vi "Check Caller.vi"(8 "error in (no error)":errorcluster, 11 "WorkSpace / Repo path":path) -> (0 "error out":errorcluster)   [LabVIEW 2019]
panel:
  out "Array 3":string[][](array[string])
  out "All Files in Dir":path[](array[path])
  out "Array":path[][](array[path])
  in  "Scan":bool
  in  "Status":string
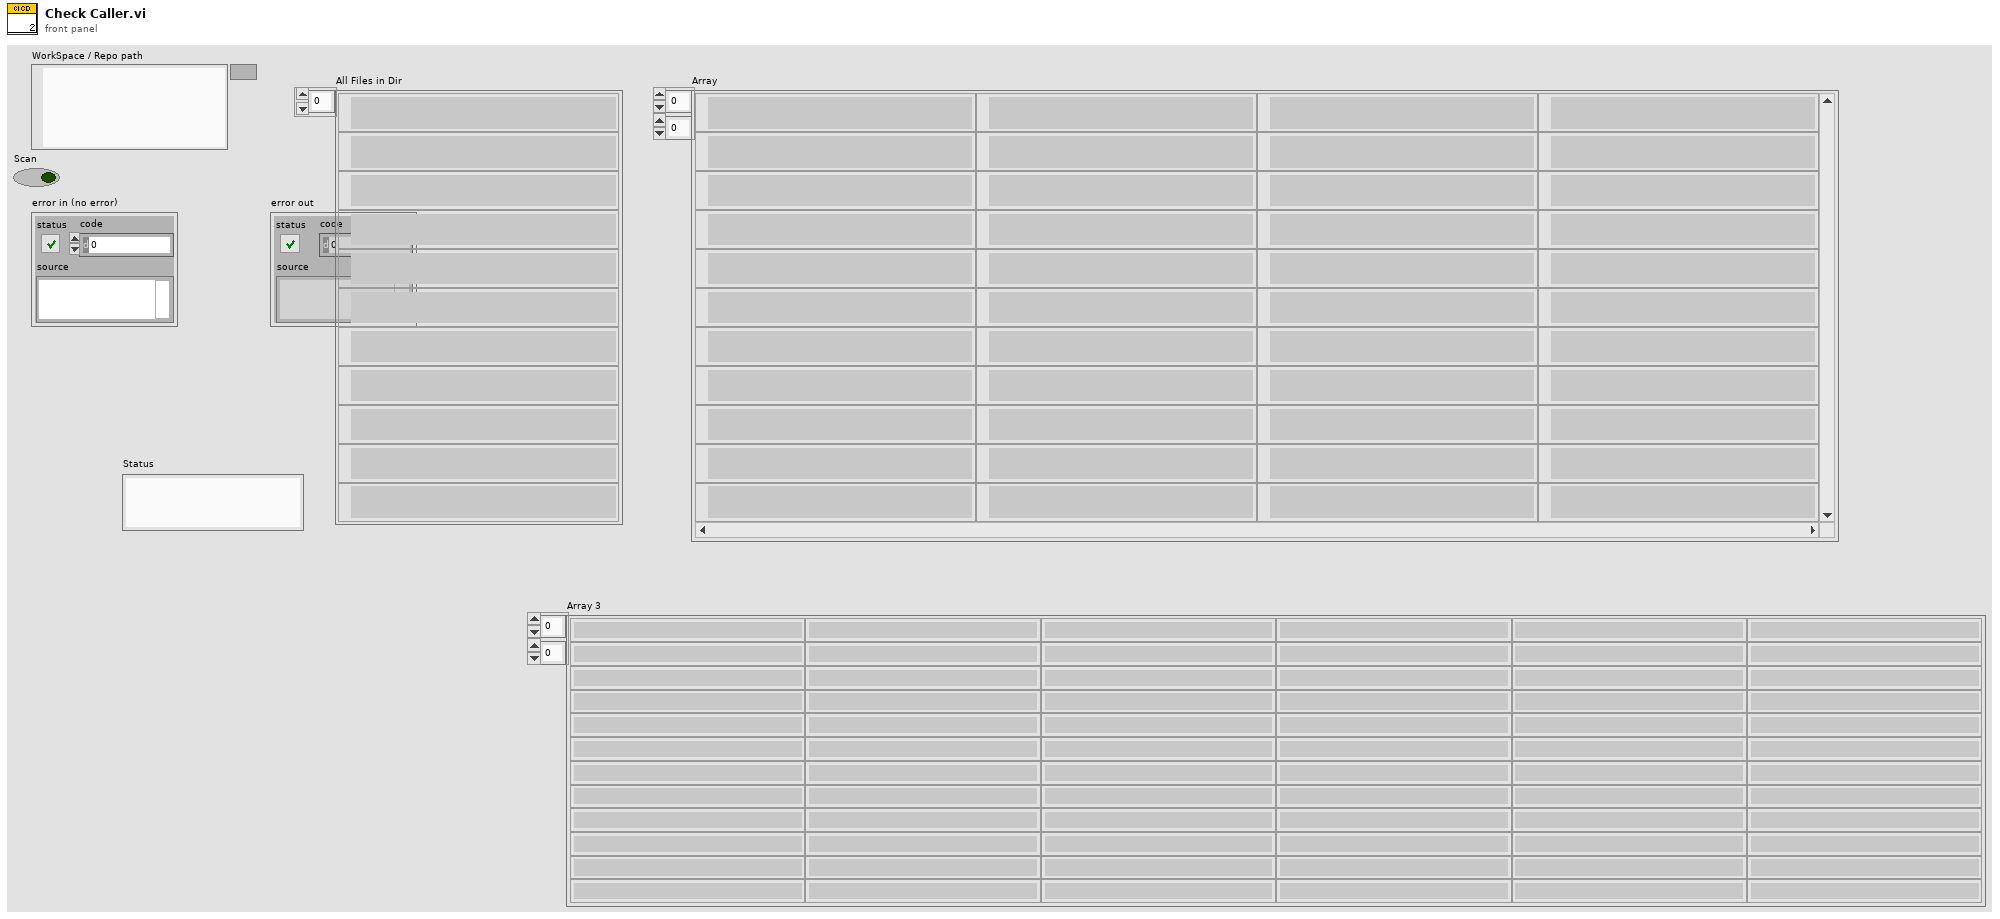
[diagram p1: front panel]
types:
  T1 = enum16{"open", "replace", "create", "open or create", "replace or create", "replace or create with confirmation"}
  T2 = typedef "NI_FileType.lvlib/LVFileType.ctl" = enum32{"Invalid file", "Unknown type", "Instrument", "Control", "Polymorphic VI", "Project", "Library", "LVClass", "XControl", "XNode", "Shared library", ".NET assembly", "ActiveX interface", "CIN", "Run-time menu", "Palette menu", "Help file", "LLB", "XNode Edit Dependency", "Class Private Data Control", "Statechart", "MathScript .m file", "Ladder Diagram", "LVLibp", "XNode Build Dependency"}
  T3 = cluster{"path":path, "delimited name":string, "type":T2, "iState":u32, "iStyle":u16, "wStyle":u16, "buttons":u16, "viflags":u32, "viflags2":u32, "links":u32[]}[]
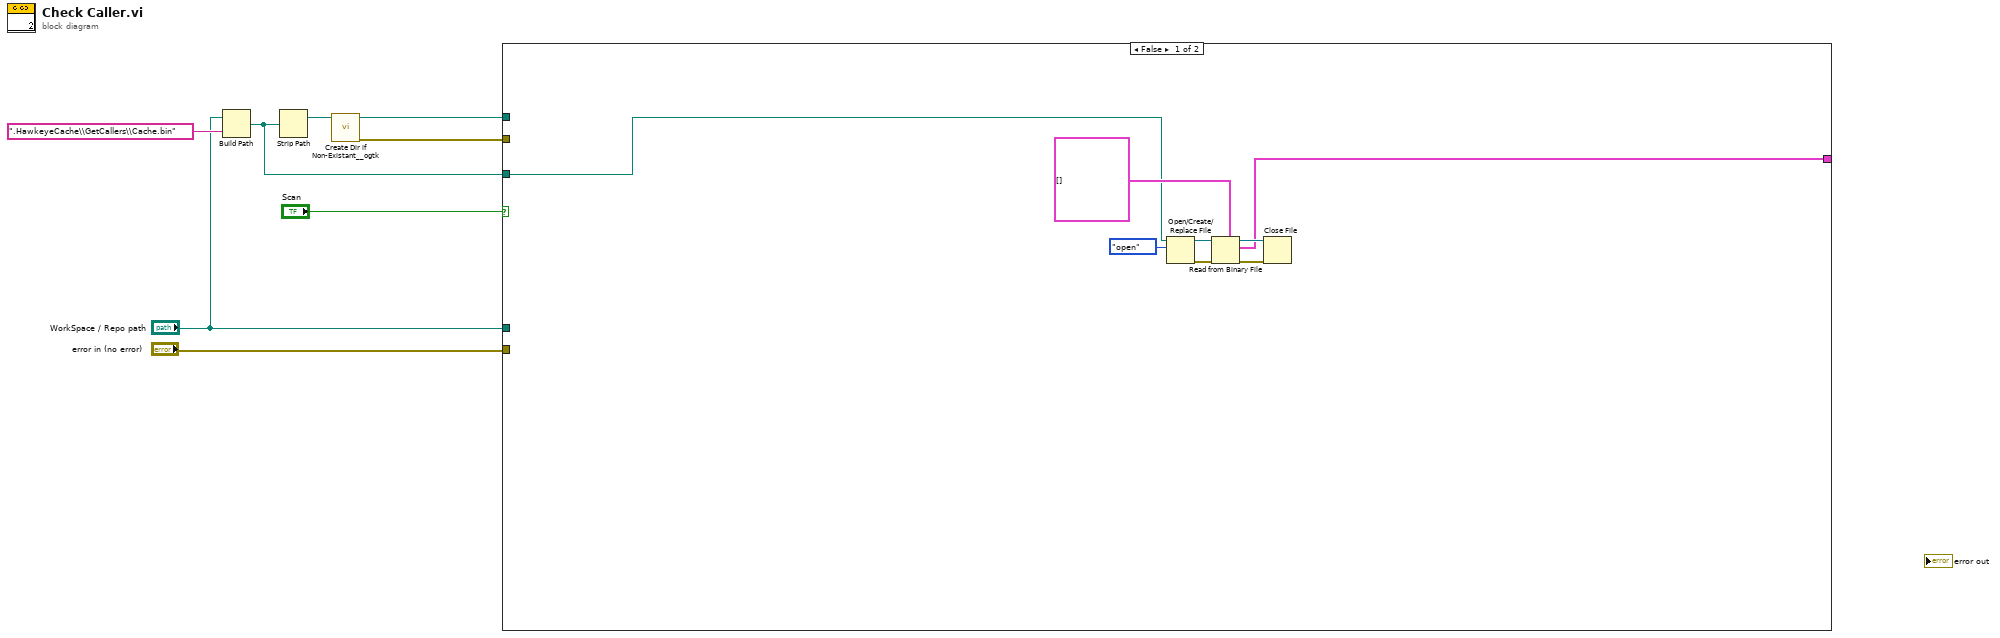
[diagram p0: block diagram]
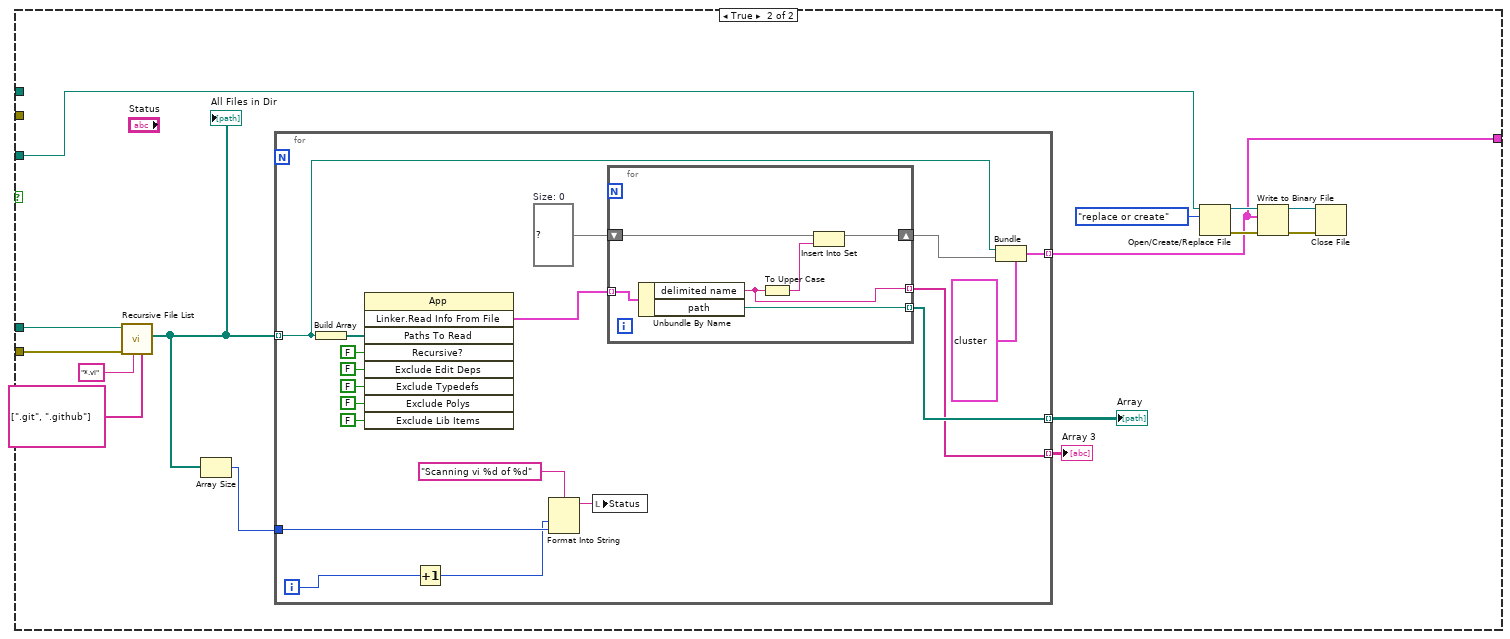
[diagram p2: hidden frame]
diagram:
  n1 = Build Path(base path="WorkSpace / Repo path", name or relative path=".HawkeyeCache\\GetCallers\\Cache.bin") -> (appended path=w1:path)
  n2 = Strip Path(path=w1) -> (stripped path=w4:path)  [unwired: 1 out]
  n3 = call <userlib>:"Create Dir if Non-Existant__ogtk.vi"("Directory Path"=w4) -> ("error out"=w3:errorcluster, "dup Directory Path"=w2:path)  [unwired: 8 in, 1 out]
  n4 = case shown="False" "Scan" {
    tunnel: "WorkSpace / Repo path" -> [_ w31]
    tunnel: "error in (no error)" -> [_ w30]
    tunnel: [w10 w20] -> _
    tunnel: w1 -> [w9 w19]
    tunnel: w3 -> [_ _]
    tunnel: w2 -> [_ _]
    frame False {
      n5 = Open/Create/Replace File(file path (use dialog)=w9, operation (0:open)=T1."open") -> (refnum out=w16:refnum<file>, error out=w12:errorcluster)  [unwired: 4 in, 1 out]
      n6 = Read from Binary File(5:cluster{"VI Path":path, "Callees":set{string}}[] [], 8:w12, 11:w16) -> (0:w14:errorcluster, 2:w10:cluster{"VI Path":path, "Callees":set{string}}[], 3:w15:refnum<file>)  [unwired: 3 in, 1 out]
      n7 = Close File(refnum=w15, error in=w14) -> ()  [unwired: 2 out]
    }
    frame True {
      n8 = call <vilib>:"Recursive File List.vi"("Folders to Exclude"=string[] [".git", ".github"], "pattern"="*.vi", "error in (no error)"=w30, "Folder Path"=w31) -> ("All Files in Dir"=w27:path[])  [unwired: 3 in, 4 out]
      "All Files in Dir" <- w27
      n9 = Array Size(array=w27) -> (size(s)=w26:i32)
      n10 = for {
        tunnel: w27 -> [w41] mode=indexing
        tunnel: w26 -> [w47]
        tunnel: [w39] -> w20 mode=indexing
        tunnel: [w37] -> w18 mode=indexing
        tunnel: [w32] -> w17 mode=indexing
        i -> [w48]
        w44 = set{string} {}  # Size: 0
        n11 = Build Array(w41) -> (w49:path[])
        n12 = invoke class="App" method="Linker.Read Info From File"("Paths To Read"=w49, "Recursive?"=FALSE, "Exclude Edit Deps"=FALSE ("Exclude Edit Time Dependencies"), "Exclude Typedefs"=FALSE, "Exclude Polys"=FALSE ("Exclude Poly VIs"), "Exclude Lib Items"=FALSE ("Exclude Unused Library Items")) -> ("Linker.Read Info From File"=w43:T3)  [unwired: 3 in, 8 out]
        n13 = Increment(x=w48) -> (x+1=w38:i32)
        n14 = Format Into String(format string="Scanning vi %d of %d", w38, w47) -> (resulting string=w45:string)  [unwired: 2 in, 1 out]
        n15 = local write "Status"(w45) -> ()
        n16 = for {
          shift-right: [w55] -> w42
          shift-left: w44 -> [w56]
          tunnel: w43 -> [w54] mode=indexing
          tunnel: [w52] -> w37 mode=indexing
          tunnel: [w51] -> w32 mode=indexing
          n17 = Unbundle By Name(w54) -> ("delimited name"=w51:string, "path"=w52:path)
          n18 = To Upper Case(1:w51) -> (0:w53:string)
          n19 = Insert Into Set(10:w53, 11:w56) -> (3:w55:set{string})  [unwired: 1 out]
        }
        n20 = Bundle(cluster=cluster{"VI Path":path, "Callees":set{string}} {"VI Path"=path "", "Callees"={}} ("output cluster"), "VI Path"=w41, "Callees"=w42) -> (w39:cluster{"VI Path":path, "Callees":set{string}})
      }
      "Array" <- w18
      "Array 3" <- w17
      n21 = Open/Create/Replace File(file path (use dialog)=w19, operation (0:open)=T1."replace or create") -> (refnum out=w24:refnum<file>, error out=w21:errorcluster)  [unwired: 4 in, 1 out]
      n22 = Write to Binary File(file (use dialog)=w24, data=w20, error in=w21) -> (refnum out=w23:refnum<file>, error out=w22:errorcluster)  [unwired: 3 in, 1 out]
      n23 = Close File(refnum=w23, error in=w22) -> ()  [unwired: 2 out]
    }
  }
